vi "Destroy.vi"(8 "error in (no error)":errorcluster, 11 "CIFFIFO in":refnum<class "CIF_CIPC_Fifo_U8.lvclass">) -> (0 "error out":errorcluster, 3 "CIFFIFO out":refnum<class "CIF_CIPC_Fifo_U8.lvclass">)   [LabVIEW 2021, in "CIF_CIPC_Fifo_U8.lvclass"]
uses:
  CIF_CIPC_Fifo_U8.lvclass
  D:/dev/Packages/CIF_Channels_Core/src/CIPC_Channels/CIF_CIPC_Chan/CIF_CIPC_Chn.lvclass
  CIF_CIPC_Chan/CIF_CIPC_Chn.lvclass/CIF_CIPC_Chn.ctl
  CIF_CIPC_Fifo_U8.lvclass/CIF_CIPC_Fifo_U8.ctl
  D:/dev/Packages/CIF_Channels_Core/src/CIFChannels/CIFChannels.lvclass
  D:/dev/Packages/CIF_Channels_Core/src/CIPC_Channels/FIFO_U8/CIF_CIPC_Fifo_U8.lvclass
  CIF_CIPC_Chan/CIF_CIPC_Chn.lvclass
  <vilib>/CIF Foundation/CIF CIPC/CIF_NI_CIPC.lvlib
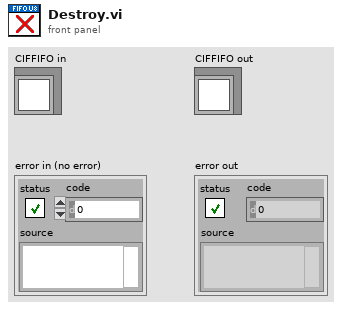
[diagram p1: front panel]
types:
  T1 = typedef "CIFChannels.lvclass/Direction.ctl" = enum16{"Publisher", "Subscriber"}
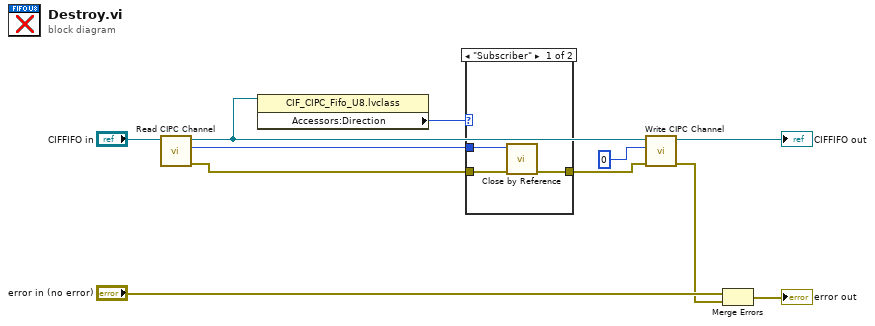
[diagram p0: block diagram]
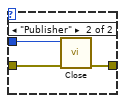
[diagram p2: hidden frame]
diagram:
  n1 = call "Read CIPC Channel.vi"("CIFTag in"="CIFFIFO in") -> ("error out"=w5:errorcluster, "CIF Channel"=w3:u64, "CIFTag out"=w2:refnum<class "CIF_CIPC_Fifo_U8.lvclass">)  [unwired: 8 in]
  n2 = property class="CIF_CIPC_Fifo_U8.lvclass"(reference=w2) -> ("Accessors:Direction"=w1:T1)  [unwired: 1 in, 2 out]
  n3 = case shown="\"Subscriber\"" w1 {
    tunnel: w5 -> [w13 w17]
    tunnel: [w12 w16] -> w4
    tunnel: w3 -> [w14 w15]
    frame "Subscriber" {
      n4 = call <vilib>:"Close by Reference.vi"("error in (no error)"=w13, "CIPC Reference"=w14) -> ("error out"=w12:errorcluster)  [unwired: 9 in]
    }
    frame "Publisher" {
      n5 = call <vilib>:"Close.vi"("error in (no error)"=w17, "CIPC Reference"=w15) -> ("error out"=w16:errorcluster)  [unwired: 9 in]
    }
  }
  n6 = call "Write CIPC Channel.vi"("error in (no error)"=w4, "CIF Channel"=u64 0, "CIFTag in"=w2) -> ("error out"=w8:errorcluster, "CIFTag out"=→"CIFFIFO out":refnum<class "CIF_CIPC_Fifo_U8.lvclass">)  [unwired: 7 in]
  n7 = Merge Errors("error in (no error)", w8) -> (→"error out":errorcluster)
